vi "Write Template.vi"(8 "error in (no error)":errorcluster, 10 "Template":string, 11 "CHEAH in":refnum<class "CHEAH.lvclass">) -> (0 "error out":errorcluster, 3 "CHEAH out":refnum<class "CHEAH.lvclass">)   [LabVIEW 2021, in "_Template.lvlib" / "CHEAH.lvclass"]
uses:
  CHEAH.lvclass
  CHEAH.lvclass/CHEAH.ctl
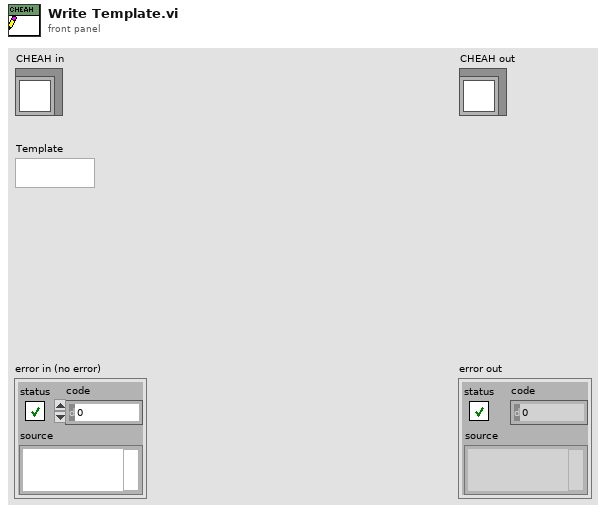
[diagram p1: front panel]
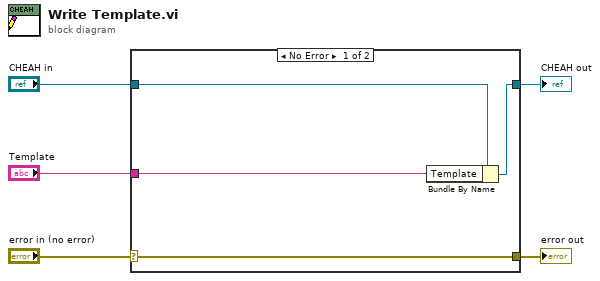
[diagram p0: block diagram]
diagram:
  n1 = case shown="No Error" "error in (no error)" {
    selector: "error in (no error)" -> [w9 w10]
    tunnel: [w9 w10] -> w4
    tunnel: [w7 w11] -> w2
    tunnel: "CHEAH in" -> [w8 w11]
    tunnel: "Template" -> [w6 _]
    frame No Error {
      n2 = Bundle By Name(cluster=w8, "Template"=w6) -> (w7:refnum<class "CHEAH.lvclass">)
    }
    frame Error {
    }
  }
  "error out" <- w4
  "CHEAH out" <- w2
